vi "Put file.vi"(8 "error in (no error)":errorcluster, 9 "Local path":path, 10 "Remote path":string, 11 "WebDAV in":refnum<class "WebDAV.lvclass">) -> (0 "error out":errorcluster, 3 "WebDAV out":refnum<class "WebDAV.lvclass">)   [LabVIEW 2015, in "RT Management.lvlib" / "WebDAV.lvclass"]
uses:
  WebDAV.lvclass
  WebDAV.lvclass/WebDAV.ctl
  Get Session.vi
  <vilib>/WebDAVClient/Advanced/Put File.vi
  <vilib>/WebDAVClient/NI_WebDAV.lvlib
  File Transfer Behavior/File Transfer Behavior.lvclass
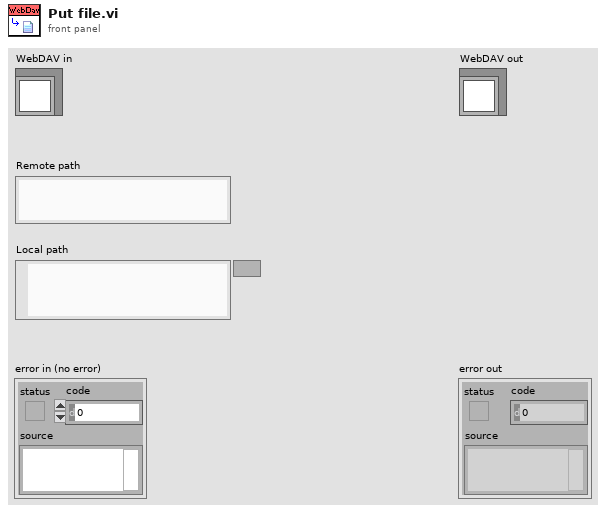
[diagram p1: front panel]
types:
  T1 = typedef "NI_WebDAV.lvlib/SessionHandle.ctl" = refnum<k1>
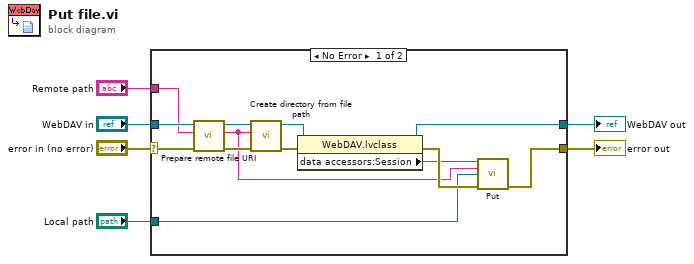
[diagram p0: block diagram]
diagram:
  n1 = case shown="No Error" "error in (no error)" {
    selector: "error in (no error)" -> [w13 w21]
    tunnel: [w16 w21] -> w5
    tunnel: "WebDAV in" -> [w14 w20]
    tunnel: [w15 w20] -> w3
    tunnel: "Remote path" -> [w7 _]
    tunnel: "Local path" -> [w17 _]
    frame No Error {
      n2 = call "Prepare remote file URI.vi"("error in (no error)"=w13, "Remote path"=w7, "WebDAV in"=w14) -> ("error out"=w12:errorcluster, "Remote file URI"=w8:string, "WebDAV out"=w11:refnum<class "WebDAV.lvclass">)  [unwired: 6 in]
      n3 = call "Create directory from file path.vi"("error in (no error)"=w12, "File path"=w8, "File Transfer Behavior in"=w11) -> ("error out"=w10:errorcluster, "File Transfer Behavior out"=w9:refnum<class "WebDAV.lvclass">)  [unwired: 7 in]
      n4 = property class="WebDAV.lvclass"(reference=w9, error in=w10) -> (reference out=w15:refnum<class "WebDAV.lvclass">, error out=w19:errorcluster, "data accessors:Session"=w18:T1)
      n5 = call-poly <vilib>:"Put.vi"("session handle"=w18, "relative uri"=w8, "local file path"=w17, "error in (no error)"=w19) -> ("error out"=w16:errorcluster)  [unwired: 9 in, 2 out]
    }
    frame Error {
    }
  }
  "error out" <- w5
  "WebDAV out" <- w3
